vi "Get stage position.vi"(4 "error in":errorcluster, 5 "input main cluster":T1) -> (0 "error out":errorcluster, 1 "output main cluster":T1, 3 "Position [micrometers]":dbl[](array[numeric]) format="%.6f")   [LabVIEW 2010]
uses:
  Main_cluster.ctl
  <vilib>/vision/Image Controls.llb/IMAQ Image.ctl
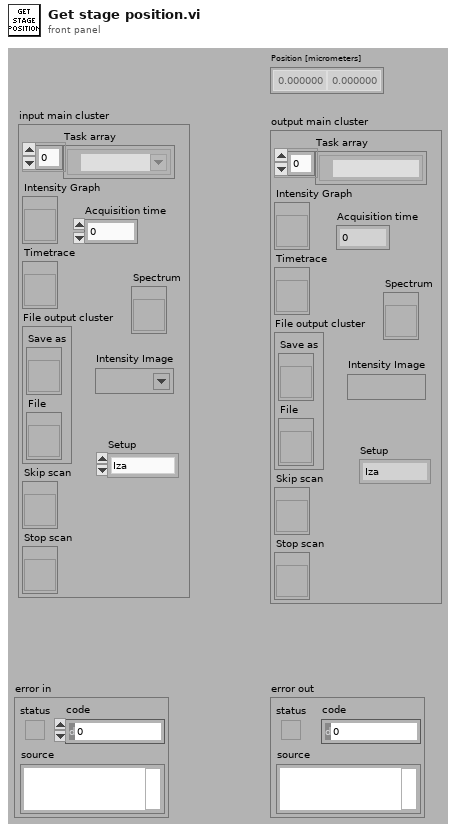
[diagram p1: front panel]
types:
  T1 = typedef "Main_cluster.ctl" = cluster{"Task array":refnum<k21>[], "Intensity Graph":refnum<vi>, "Timetrace":refnum<vi>, "File output cluster":cluster{"Save as":refnum<vi>, "File":refnum<vi>}, "Skip scan":refnum<vi>, "Stop scan":refnum<vi>, "Acquisition time":dbl, "Setup":enum16{"Iza", "Lukasz"}, "Spectrum":refnum<vi>, "Intensity Image":T2}
  T2 = typedef "IMAQ Image.ctl" = refnum<image>
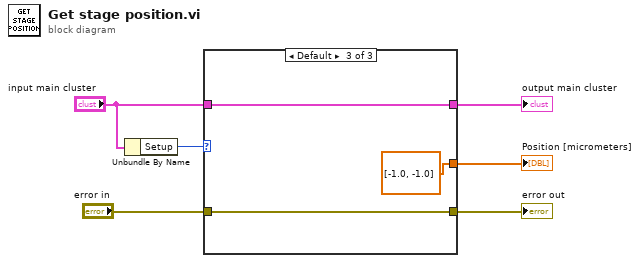
[diagram p0: block diagram]
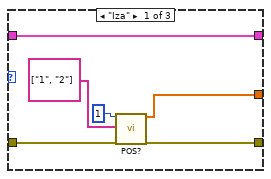
[diagram p2: hidden frame]
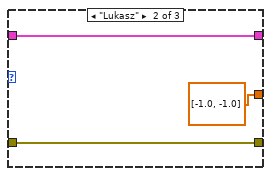
[diagram p3: hidden frame]
diagram:
  n1 = Unbundle By Name("input main cluster") -> ("Setup"=w3:enum16{"Iza", "Lukasz"})
  n2 = case shown="Default" w3 {
    tunnel: [w12 dbl[] [-1.0, -1.0] ("Position") dbl[] [-1.0, -1.0] ("Position")] -> w6
    tunnel: [w9 w14 w17] -> w5
    tunnel: "error in" -> [w8 w14 w17]
    tunnel: "input main cluster" -> [w7 w15 w18]
    tunnel: [w7 w15 w18] -> w1
    frame "Iza" {
      n3 = call "POS?.vi"("System no."=1, "Axes to query"=string[] ["1", "2"], "error in"=w8) -> ("Position"=w12:dbl[], "error out"=w9:errorcluster)  [unwired: 15 in]
    }
    frame "Lukasz" {
    }
    frame Default {
    }
  }
  "Position [micrometers]" <- w6
  "error out" <- w5
  "output main cluster" <- w1
